vi "Add Response (Server Error from Request).vi"(6 "code (-32000 to -32099)":i32=-32000, 7 "Request":refnum<class "Request.lvclass">, 8 "error in (no error)":errorcluster, 10 "data":variant, 11 "Server in":refnum<class "JSONRPC Server.lvclass">) -> (0 "error out":errorcluster, 1 "response string":string, 3 "Server out":refnum<class "JSONRPC Server.lvclass">)   [LabVIEW 2020, in "JSON-RPC Lib.lvlib" / "JSONRPC Server.lvclass"]
uses:
  JSONRPC Server.lvclass
  Request/Request.lvclass
  Request/Request.lvclass/Request.ctl
  Request/request.Read jsonrpc.vi
  Request/request.Read id value.vi
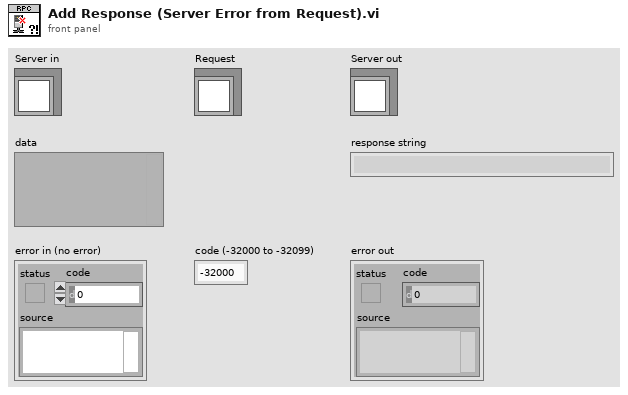
[diagram p1: front panel]
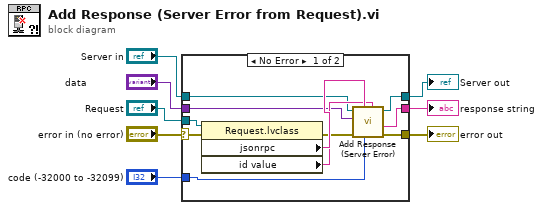
[diagram p0: block diagram]
diagram:
  n1 = case shown="No Error" "error in (no error)" {
    selector: "error in (no error)" -> [w19 w21]
    tunnel: [w12 w21] -> w7
    tunnel: [w14 w20] -> w5
    tunnel: "Server in" -> [w15 w20]
    tunnel: "Request" -> [w18 _]
    tunnel: "data" -> [w11 _]
    tunnel: "code (-32000 to -32099)" -> [w10 _]
    tunnel: [w9 _] -> w1
    frame No Error {
      n2 = property class="Request.lvclass"(reference=w18, error in=w19) -> (error out=w13:errorcluster, "jsonrpc"=w17:string, "id value"=w16:string)  [unwired: 1 out]
      n3 = call "Add Response (Server Error).vi"("id value"=w16, "code (-32000 to -32099)"=w10, "jsonrpc"=w17, "error in (no error)"=w13, "data"=w11, "Server in"=w15) -> ("error out"=w12:errorcluster, "response string"=w9:string, "Server out"=w14:refnum<class "JSONRPC Server.lvclass">)  [unwired: 3 in]
    }
    frame Error {
    }
  }
  "error out" <- w7
  "Server out" <- w5
  "response string" <- w1
